vi "registerClouds_PCL.vi"(0 "cloudX_target":sgl[](array[numeric])=[1.05222, 0.302594, -0.0318983, -0.0347655, 0.2393], 1 "cloudY_target":sgl[](array[numeric])=[-0.151883, -0.473106, 0.667105, 0.854581, -0.277468], 3 "icp_max_correspondence_distance":dbl=0.5, 4 "icp_transformation_epsilon":dbl=1e-10, 5 "cloudZ_target":sgl[](array[numeric])=[-0.106395, 0.292602, 0.441304, -0.0361733, -0.916762], 6 "isDense":bool, 7 "cloudX_source":sgl[](array[numeric])=[0.352222, -0.397406, -0.731898, -0.734766, -0.4607], 8 "icp_ransac_threshold":dbl=0.5, 9 "cloudY_source":sgl[](array[numeric])=[-0.151883, -0.473106, 0.667105, 0.854581, -0.277468], 10 "registration type\n(0 full, < 0 icp only, > 0 sac-ia only)":i32, 11 "ia_maximum_iterations":i32=100, 12 "ia_max_correspondence_distance":sgl=0.5, 13 "icp_euclidean_fitness_epsilon":dbl=1e-08, 14 "ia_min_sample_distance":sgl=0.01, 16 "icp_max_iterations":i32=100, 17 "cloudZ_source":sgl[](array[numeric])=[-0.106395, 0.292602, 0.441304, -0.0361733, -0.916762], 18 "normals_radius":dbl=0.015 format="%#_13g", 19 "fpfh_radius":dbl=0.03 format="%#_13g") -> (15 "rotation matrix":sgl[][](array[numeric])=[[1.0000002, 2.1462839e-07, -1.6423296e-07], [-1.3767561e-07, 1.0, -6.5921284e-08], [1.6773438e-07, 2.9214991e-08, 1.0]], 20 "transformation_matrix":sgl[][](array[numeric])=[[1.0000002, 2.1462839e-07, -1.6423296e-07, 0.7000001], [-1.3767561e-07, 1.0, -6.5921284e-08, -7.4505806e-08], [1.6773438e-07, 2.9214991e-08, 1.0, 9.313226e-08], [0.0, 0.0, 0.0, 1.0]], 21 "score":dbl=1.0883044465614945e-12, 24 "processing time [ms]":u32=43, 25 "converged?":bool=TRUE, 27 "translation vector":sgl[](array[numeric])=[0.7000001, -7.4505806e-08, 9.313226e-08])   [LabVIEW 2012]
uses:
  dlls/PCL_OpenCV_LabviewToolkit.dll
panel:
  out "Rz angle [rad]":sgl=-1.3767558e-07
  out "Rx angle [rad]":sgl=2.9214991e-08
  out "Ry angle [rad]":sgl=-1.6773438e-07
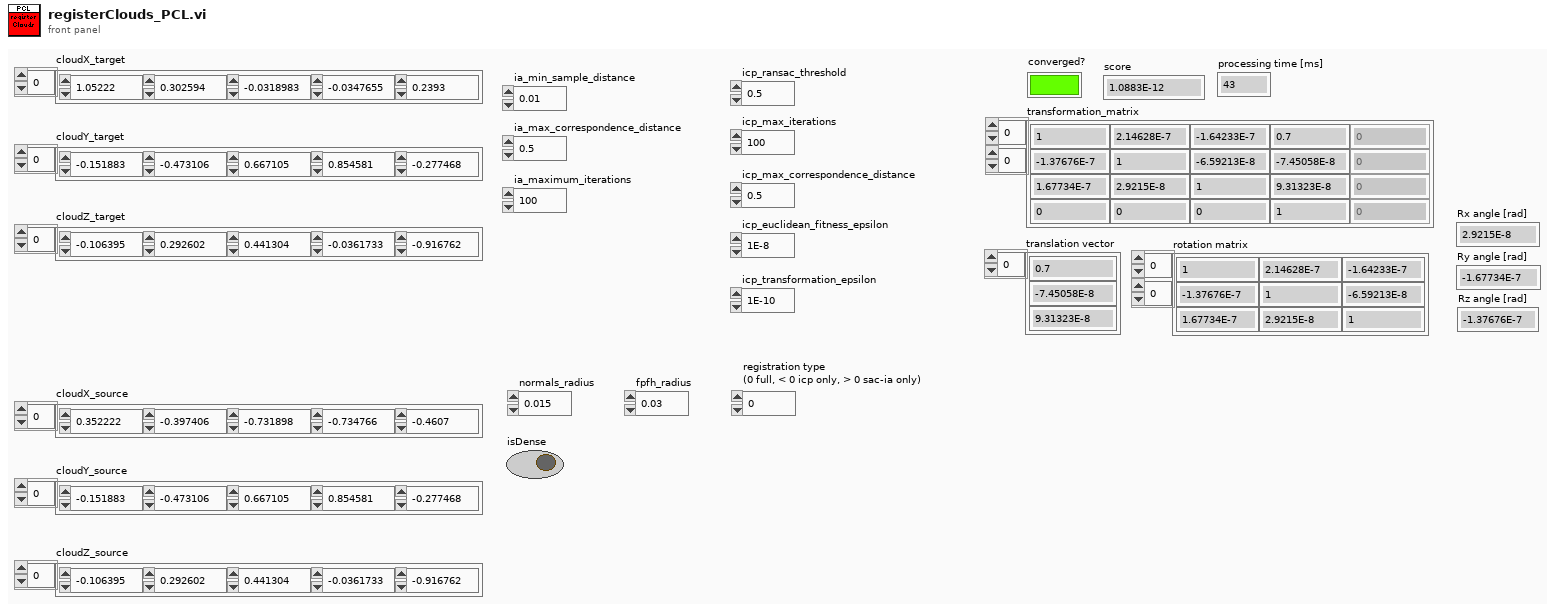
[diagram p1: front panel]
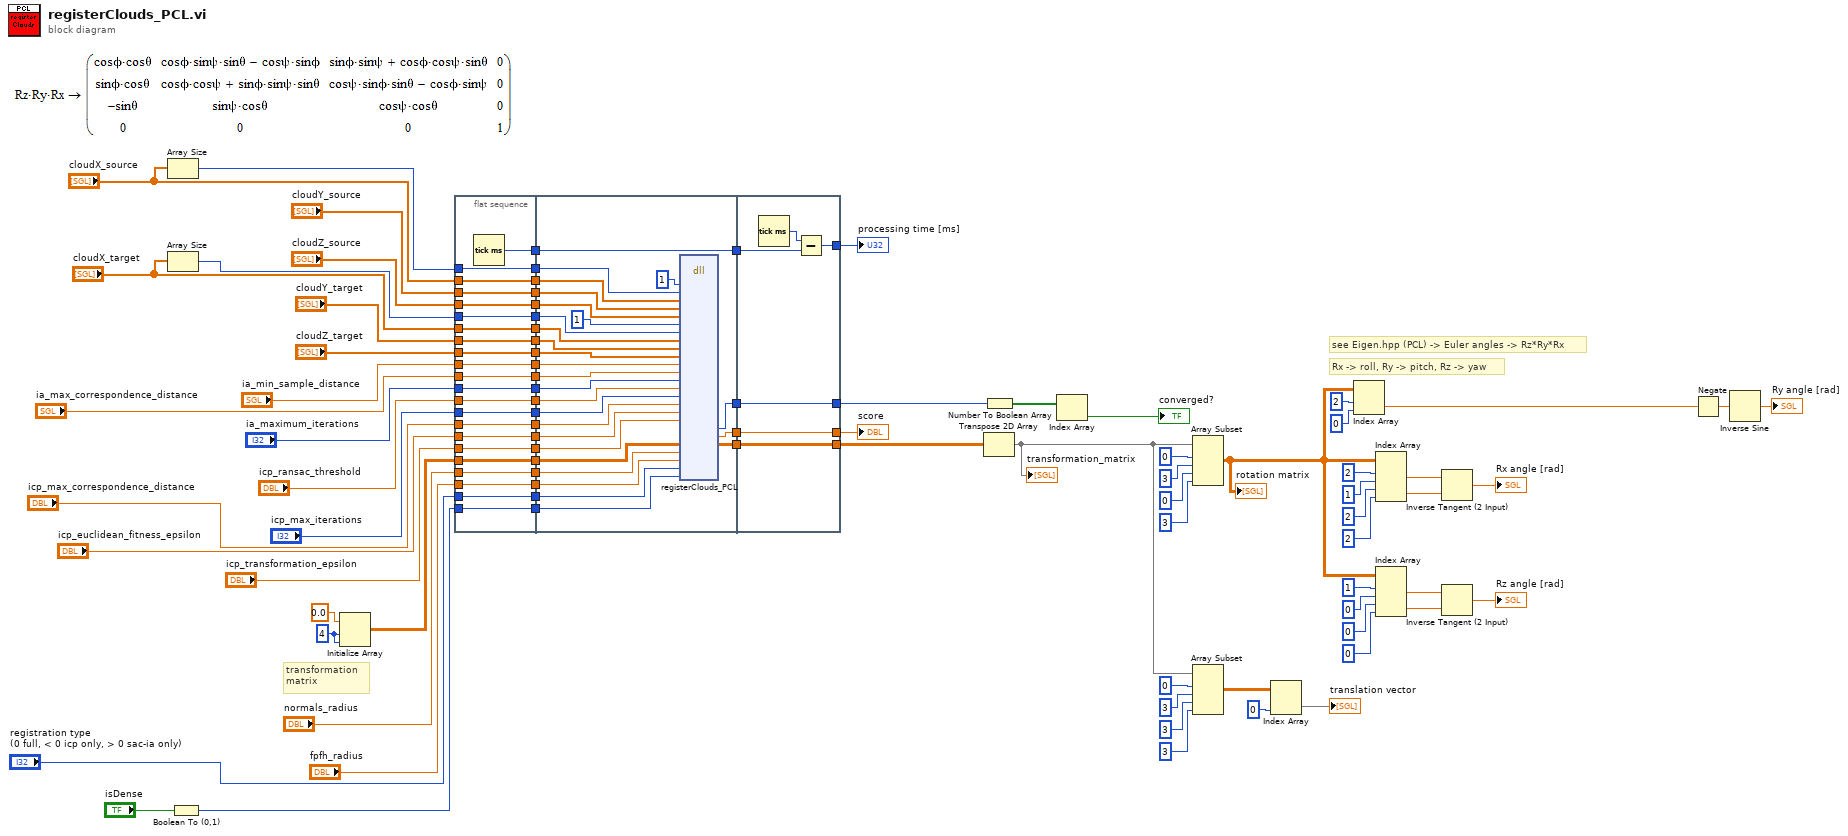
[diagram p0: block diagram]
diagram:
  w81 = 4 ("dimension size")
  # "Rx -> roll, Ry -> pitch, Rz -> yaw"
  # "see Eigen.hpp (PCL) -> Euler angles -> Rz*Ry*Rx"
  # "transformation \nmatrix"
  n1 = Array Size(array="cloudX_source") -> (size(s)=w2:i32)
  n2 = Array Size(array="cloudX_target") -> (size(s)=w1:i32)
  n3 = Boolean To (0,1)(Boolean="isDense") -> (0, 1=w4:i16)
  n4 = Initialize Array(sgl 0.0 ("element"), w81, w81) -> (w24:sgl[][])
  n5 = flat-sequence {
    tunnel: "icp_max_iterations" -> [w99]
    tunnel: "icp_ransac_threshold" -> [w100]
    tunnel: "cloudZ_source" -> [w107]
    tunnel: "cloudY_source" -> [w108]
    tunnel: "cloudX_source" -> [w109]
    tunnel: [w110] -> w74
    tunnel: "icp_max_correspondence_distance" -> [w98]
    tunnel: "icp_euclidean_fitness_epsilon" -> [w97]
    tunnel: "icp_transformation_epsilon" -> [w96]
    tunnel: [w109] -> w35
    tunnel: [w108] -> w34
    tunnel: [w107] -> w33
    tunnel: w2 -> [w106]
    tunnel: [w106] -> w32
    tunnel: "cloudX_target" -> [w105]
    tunnel: [w105] -> w31
    tunnel: "cloudY_target" -> [w104]
    tunnel: [w104] -> w29
    tunnel: "cloudZ_target" -> [w103]
    tunnel: [w103] -> w27
    tunnel: w1 -> [w102]
    tunnel: [w102] -> w25
    tunnel: w24 -> [w101]
    tunnel: [w101] -> w23
    tunnel: [w100] -> w22
    tunnel: [w99] -> w21
    tunnel: [w98] -> w20
    tunnel: [w97] -> w19
    tunnel: [w96] -> w18
    tunnel: "ia_min_sample_distance" -> [w95]
    tunnel: [w95] -> w16
    tunnel: "ia_max_correspondence_distance" -> [w94]
    tunnel: [w94] -> w14
    tunnel: "ia_maximum_iterations" -> [w93]
    tunnel: [w93] -> w12
    tunnel: "normals_radius" -> [w92]
    tunnel: [w92] -> w10
    tunnel: "fpfh_radius" -> [w91]
    tunnel: [w91] -> w8
    tunnel: "registration type\n(0 full, < 0 icp only, > 0 sac-ia only)" -> [w90]
    tunnel: [w90] -> w6
    tunnel: w4 -> [w89]
    tunnel: [w89] -> w3
    tunnel: [w137] -> w77
    tunnel: [w136] -> w76
    tunnel: [w135] -> w75
    tunnel: w74 -> [w134]
    tunnel: [w134] -> w73
    tunnel: w35 -> [w133]
    tunnel: w34 -> [w132]
    tunnel: w33 -> [w131]
    tunnel: w32 -> [w130]
    tunnel: w31 -> [w129]
    tunnel: w29 -> [w128]
    tunnel: w27 -> [w127]
    tunnel: w25 -> [w126]
    tunnel: w23 -> [w125]
    tunnel: w22 -> [w124]
    tunnel: w21 -> [w123]
    tunnel: w20 -> [w122]
    tunnel: w19 -> [w121]
    tunnel: w18 -> [w120]
    tunnel: w16 -> [w119]
    tunnel: w14 -> [w118]
    tunnel: w12 -> [w117]
    tunnel: w10 -> [w116]
    tunnel: w8 -> [w115]
    tunnel: w6 -> [w114]
    tunnel: w3 -> [w113]
    tunnel: [w141] -> w80
    tunnel: [w142] -> w83
    tunnel: [w143] -> w85
    tunnel: w77 -> [w143]
    tunnel: w76 -> [w142]
    tunnel: w75 -> [w141]
    tunnel: w73 -> [w140]
    tunnel: [w138] -> w72
    frame #0 {
      n6 = Tick Count (ms)() -> (millisecond timer value=w110:u32)
    }
    frame #1 {
      n7 = dll-call lib="C:/eurecar/3d/dlls/PCL_OpenCV_LabviewToolkit.dll" fn="registerClouds_PCL"("cloudCols_source"=1, "cloudRows_source"=w130, "cloudX_source"=w133, "cloudY_source"=w132, "cloudZ_source"=w131, "cloudCols_target"=1, "cloudRows_target"=w126, "cloudX_target"=w129, "cloudY_target"=w128, "cloudZ_target"=w127, "ia_min_sample_distance"=w119, "ia_max_correspondence_distance"=w118, "ia_maximum_iterations"=w117, "icp_ransac_threshold"=w124, "icp_max_iterations"=w123, "icp_max_orrespondence_distance"=w122, "icp_euclidean_fitness_epsilon"=w121, "icp_transformation_epsilon"=w120, "final_transformation_matrix"=w125, "normals_radius"=w116, "fpfh_radius"=w115, "registration_type"=w114, "dense"=w113) -> ("icp_converged"=w137:i32, "icp_score"=w136:dbl, "final_transformation_matrix"=w135:sgl[][])  [unwired: 28 in, 2 out]
    }
    frame #2 {
      n8 = Tick Count (ms)() -> (millisecond timer value=w139:u32)
      n9 = Subtract(x=w139, y=w140) -> (x-y=w138:u32)
    }
  }
  n10 = Transpose 2D Array(2D array=w80) -> (transposed array=w71:sgl[][])
  "transformation_matrix" <- w71
  n11 = Number To Boolean Array(number=w85) -> (Boolean array=w86:bool[])
  n12 = Index Array(array=w86) -> (element=→"converged?":bool)  [unwired: 1 in]
  n13 = Array Subset(array=w71, index (row)=0 ("index"), length (row)=3 ("index"), index (col)=0 ("index"), length (col)=3 ("index")) -> (w43:sgl[][])
  "rotation matrix" <- w43
  n14 = Array Subset(array=w71, index (row)=0 ("index"), length (row)=3 ("index"), index (col)=3 ("index"), length (col)=3 ("index")) -> (w66:sgl[][])
  n15 = Index Array(array=w66, index (col)=0 ("disabled index (col)")) -> (element=→"translation vector":sgl[])  [unwired: 1 in]
  n16 = Index Array(array=w43, index (row)=2, index (col)=0 ("disabled index (col)")) -> (element=w57:sgl)
  n17 = Index Array(array=w43, index (row) #1=2 ("index (row)"), index (col) #1=1 ("disabled index (col)"), index (row) #2=2 ("index (row)"), index (col) #2=2 ("index (row)")) -> (element #1=w51:sgl, element #2=w50:sgl)
  n18 = Index Array(array=w43, index (row) #1=1 ("index (row)"), index (col) #1=0 ("disabled index (col)"), index (row) #2=0 ("index (row)"), index (col) #2=0 ("index (row)")) -> (element #1=w48:sgl, element #2=w49:sgl)
  n19 = Inverse Tangent (2 Input)(1:w50, 2:w51) -> (0:→"Rx angle [rad]":sgl)
  n20 = Inverse Tangent (2 Input)(1:w49, 2:w48) -> (0:→"Rz angle [rad]":sgl)
  n21 = Negate(x=w57) -> (-x=w56:sgl)
  n22 = Inverse Sine(1:w56) -> (0:→"Ry angle [rad]":sgl)
  "score" <- w83
  "processing time [ms]" <- w72
